vi "Proxy_Build VI Package_vipm_api.vi"(8 "error in (no error)":errorcluster, 10 "Path to VIPB File":path) -> (0 "error out":errorcluster, 2 "Build Output":path)   [LabVIEW 2017, in "CL_G3_VIPMUtilities.lvlib"]
doc: "This VI dynamically invokes the VIPM API with a timeout. VPIM will randomly hang for reasons we don't understand. This vi detects if there is a hang, force closes VIPM and then restarts it."
uses:
  CL_G3_VIPMUtilities.lvlib
  Proxy States.ctl
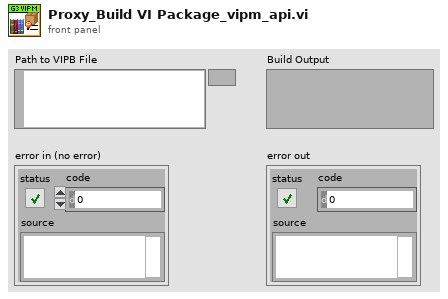
[diagram p1: front panel]
types:
  T1 = typedef "CL_G3_VIPMUtilities.lvlib/Proxy States.ctl" = enum16{"Initialize", "Start Proxy", "Wait on Proxy", "Force Quit VIPM", "Close Proxy"}
  T2 = cluster{"Proxy Path":path, "error out":errorcluster, "Proxy VI Ref":refnum<vi>, "Restart Count":i32, "Maximum restart tries":i32, "Path to VIPB File":path, "Build Output":path}
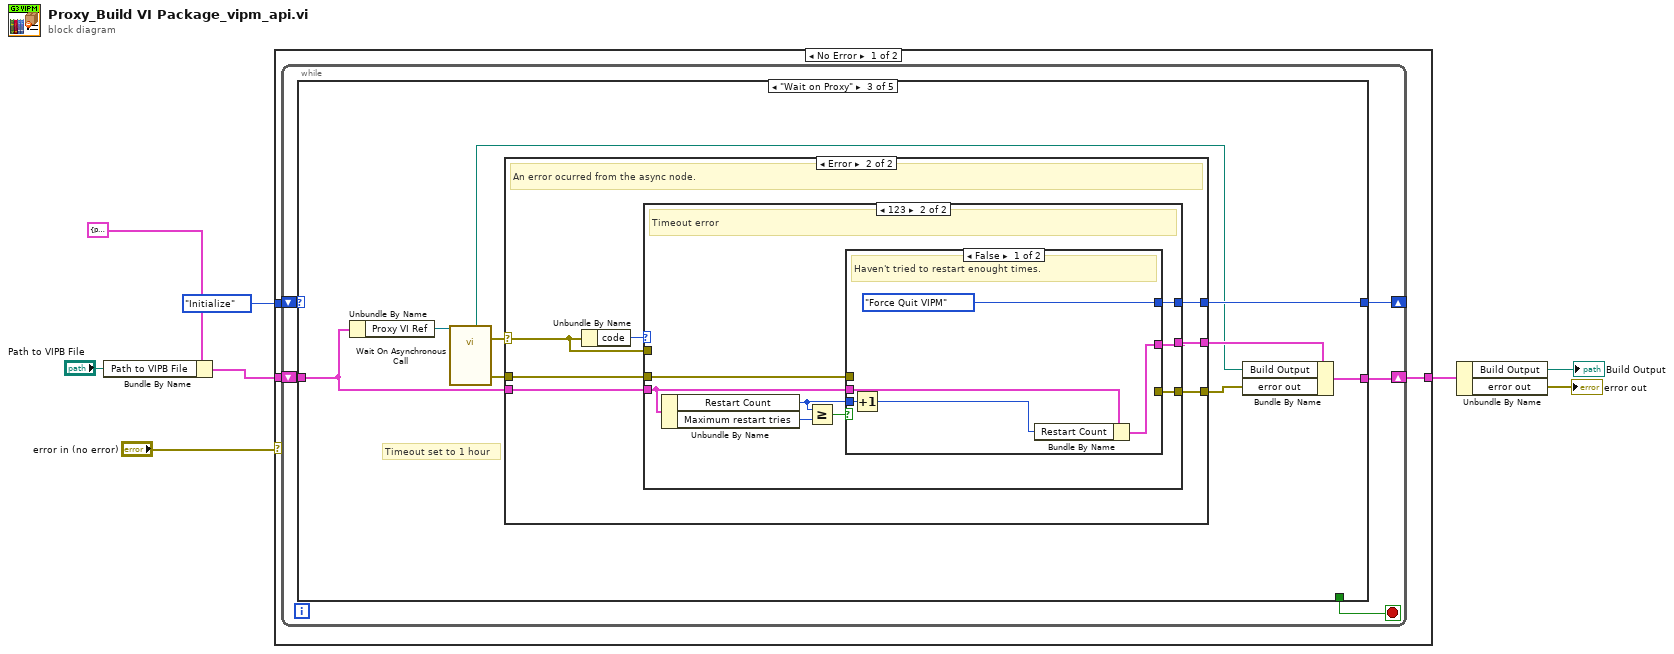
[diagram p0: block diagram]
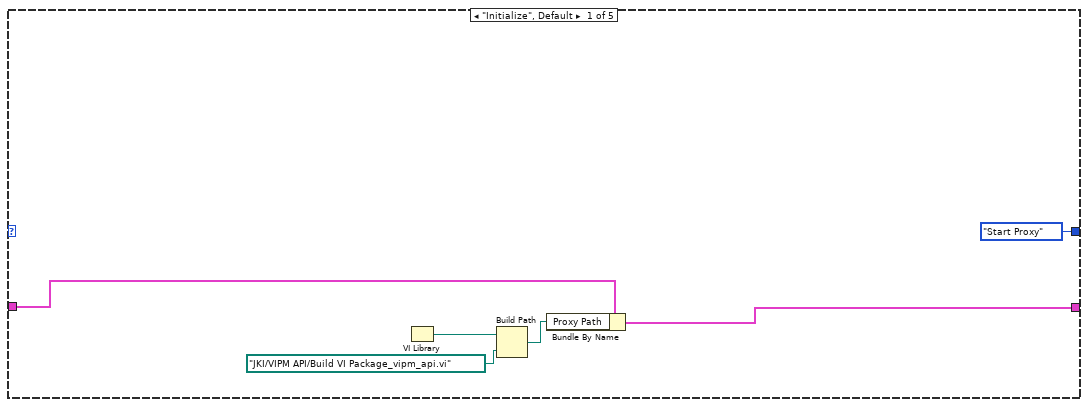
[diagram p2: hidden frame]
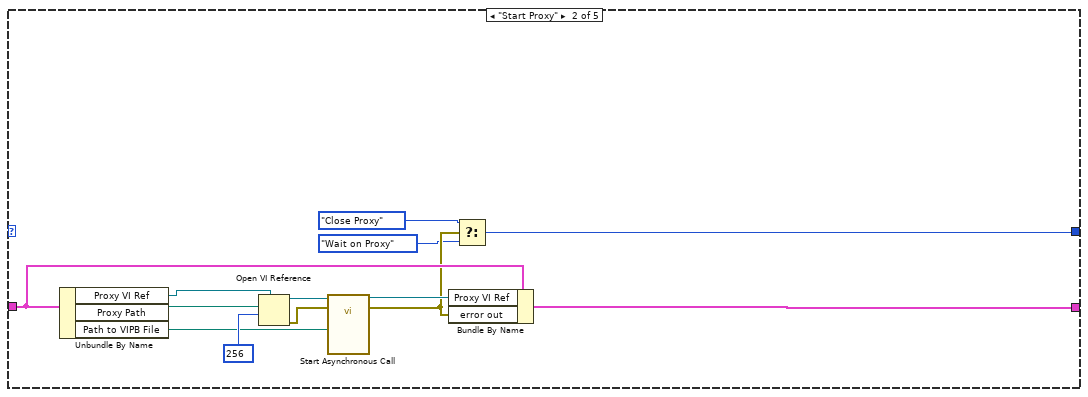
[diagram p3: hidden frame]
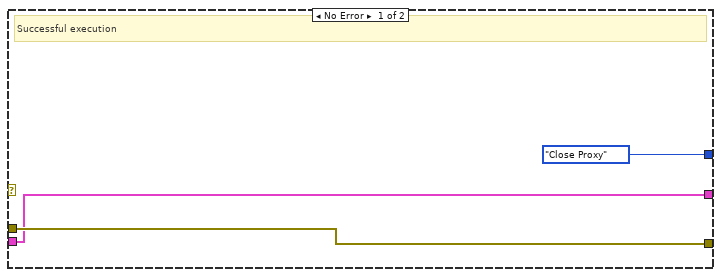
[diagram p4: hidden frame]
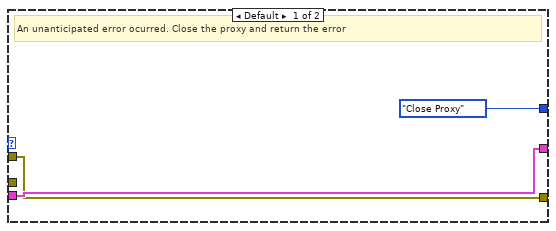
[diagram p5: hidden frame]
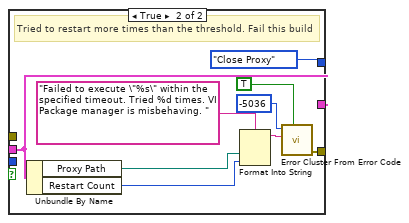
[diagram p6: hidden frame]
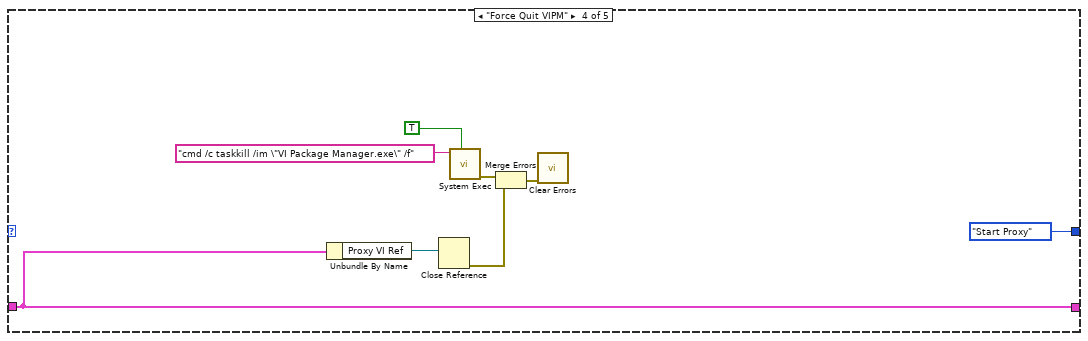
[diagram p7: hidden frame]
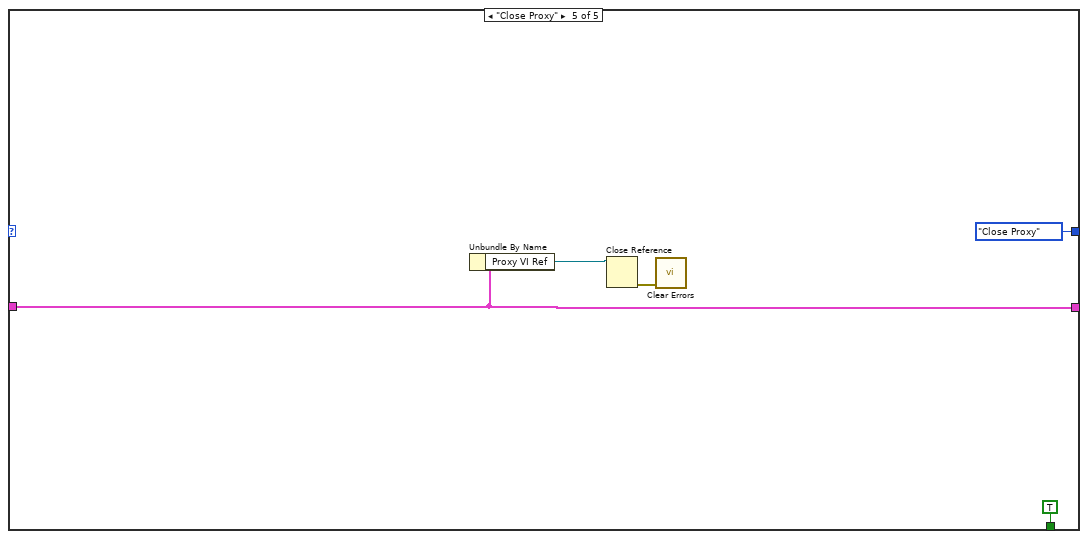
[diagram p8: hidden frame]
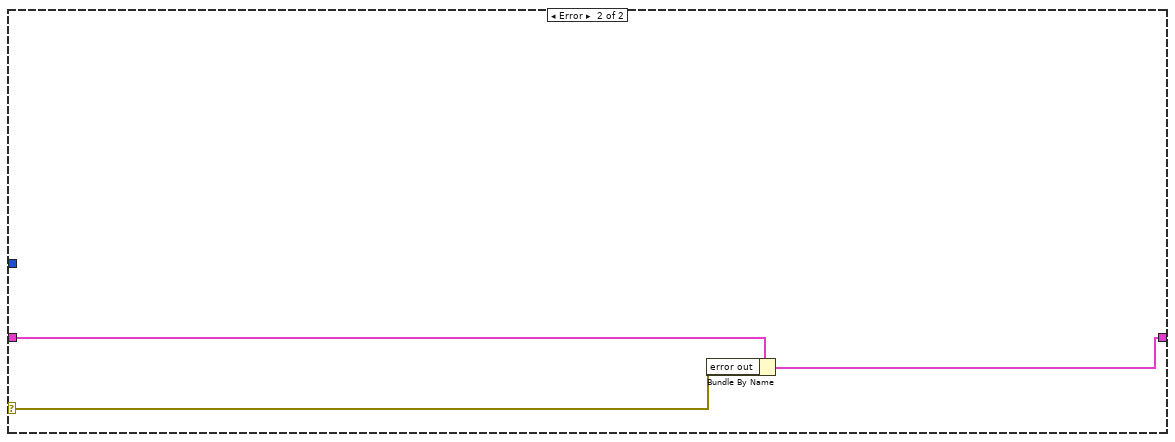
[diagram p9: hidden frame]
diagram:
  n1 = Bundle By Name(cluster=T2 {"Proxy Path"=path "", "error out"={"status"=FALSE, "code"=0, "source"=""}, "Proxy VI Ref"=refnum, "Restart Count"=0, "Maximum restart tries"=5, "Path to VIPB File"=path "", "Build Output"=path ""}, "Path to VIPB File"="Path to VIPB File") -> (w7:T2)
  n2 = case shown="No Error" "error in (no error)" {
    selector: "error in (no error)" -> [_ w94]
    tunnel: w7 -> [w11 w95]
    tunnel: Proxy_States."Initialize" -> [w10 _]
    tunnel: [w9 w93] -> w4
    frame No Error {
      n3 = while {
        shift-right: [w14] -> _
        shift-left: w10 -> [w16]
        shift-right: [w13] -> w9
        shift-left: w11 -> [w15]
        stop <- w12 stop-if-true
        n4 = case shown="\"Wait on Proxy\"" w16 {
          tunnel: [w21 w31 w44 w83 w90] -> w13
          tunnel: w15 -> [w22 w35 w40 w83 w90]
          tunnel: [Proxy_States."Start Proxy" w26 w38 Proxy_States."Start Proxy" Proxy_States."Close Proxy"] -> w14
          tunnel: [_ _ _ _ TRUE] -> w12
          frame "Initialize", Default {
            n5 = VI Library() -> (path=w19:path)
            n6 = Build Path(base path=w19, name or relative path=path "JKI/VIPM API/Build VI Package_vipm_api.vi" ("Proxy Path")) -> (appended path=w17:path)
            n7 = Bundle By Name(cluster=w22, "Proxy Path"=w17) -> (w21:T2)
          }
          frame "Start Proxy" {
            n8 = Unbundle By Name(w35) -> ("Proxy VI Ref"=w25:refnum<vi>, "Proxy Path"=w34:path, "Path to VIPB File"=w23:path)
            n9 = Open VI Reference(type specifier VI Refnum (for type only)=w25, vi path=w34, options=256) -> (vi reference=w33:refnum<vi>, error out=w32:errorcluster)  [unwired: 3 in]
            n10 = call-by-ref "Start Asynchronous Call"(reference=w33, error in=w32, "Path to VIPB File"=w23) -> (reference out=w30:refnum<vi>, error out=w29:errorcluster)  [unwired: 9 in, 2 out]
            n11 = Bundle By Name(cluster=w35, "Proxy VI Ref"=w30, "error out"=w29) -> (w31:T2)
            n12 = Select(t=Proxy_States."Close Proxy", s=w29, f=Proxy_States."Wait on Proxy") -> (s? t:f=w26:T1)
          }
          frame "Wait on Proxy" {
            # "Timeout set to 1 hour"
            n13 = Unbundle By Name(w40) -> ("Proxy VI Ref"=w36:refnum<vi>)
            n14 = call-by-ref "Wait On Asynchronous Call"(reference=w36) -> (error out=w41:errorcluster, 0:"error out"=w42:errorcluster, "Build Output"=w37:path)  [unwired: 11 in, 1 out]
            n15 = case shown="Error" w41 {
              selector: w41 -> [_ w48]
              tunnel: [w47 w51] -> w43
              tunnel: w42 -> [w47 w50]
              tunnel: w40 -> [w45 w53]
              tunnel: [w45 w52] -> w39
              tunnel: [Proxy_States."Close Proxy" w49] -> w38
              frame No Error {
                # "Successful execution"
              }
              frame Error {
                # "An error ocurred from the async node."
                n16 = Unbundle By Name(w48) -> ("code"=w54:i32)
                n17 = case shown="123" w54 {
                  tunnel: w53 -> [w57 w65]
                  tunnel: [w57 w64] -> w52
                  tunnel: [w55 w60] -> w51
                  tunnel: w50 -> [_ w59]
                  tunnel: [Proxy_States."Close Proxy" w61] -> w49
                  tunnel: w48 -> [w55 _]
                  frame Default {
                    # "An unanticipated error ocurred. Close the proxy and return the error"
                  }
                  frame 123 {
                    # "Timeout error"
                    n18 = Unbundle By Name(w65) -> ("Restart Count"=w63:i32, "Maximum restart tries"=w58:i32)
                    n19 = Greater Or Equal?(x=w63, y=w58) -> (x >= y?=w62:bool)
                    n20 = case shown="False" w62 {
                      tunnel: w65 -> [w70 w73]
                      tunnel: [w69 w73] -> w64
                      tunnel: w63 -> [w66 _]
                      tunnel: [Proxy_States."Force Quit VIPM" Proxy_States."Close Proxy"] -> w61
                      tunnel: [_ w77] -> w60
                      tunnel: w59 -> [_ _]
                      frame False {
                        # "Haven't tried to restart enought times."
                        n21 = Increment(x=w66) -> (x+1=w67:i32)
                        n22 = Bundle By Name(cluster=w70, "Restart Count"=w67) -> (w69:T2)
                      }
                      frame True {
                        # "Tried to restart more times than the threshold. Fail this build"
                        n23 = Unbundle By Name(w73) -> ("Proxy Path"=w72:path, "Restart Count"=w71:i32)
                        n24 = Format Into String(format string="Failed to execute \"%s\" within the specified timeout. Tried %d times. VI Package manager is misbehaving. ", w72, w71) -> (resulting string=w74:string)  [unwired: 2 in, 1 out]
                        n25 = call <vilib>:"Error Cluster From Error Code.vi"("show call chain? (False)"=TRUE, "error message (\"\")"=w74, "error code (0)"=-5036) -> ("error out"=w77:errorcluster)  [unwired: 6 in]
                      }
                    }
                  }
                }
              }
            }
            n26 = Bundle By Name(cluster=w39, "Build Output"=w37, "error out"=w43) -> (w44:T2)
          }
          frame "Force Quit VIPM" {
            n27 = Unbundle By Name(w83) -> ("Proxy VI Ref"=w82:refnum<vi>)
            n28 = Close Reference(reference=w82) -> (error out=w80:errorcluster)  [unwired: 1 in]
            n29 = call <vilib>:"System Exec.vi"("run minimized? (F)"=TRUE, "command line"="cmd /c taskkill /im \"VI Package Manager.exe\" /f") -> ("error out"=w85:errorcluster)  [unwired: 6 in, 3 out]
            n30 = Merge Errors(w85, w80) -> (w81:errorcluster)
            n31 = call <vilib>:"Clear Errors.vi"("error in (no error)"=w81) -> ()  [unwired: 5 in, 2 out]
          }
          frame "Close Proxy" {
            n32 = Unbundle By Name(w90) -> ("Proxy VI Ref"=w89:refnum<vi>)
            n33 = Close Reference(reference=w89) -> (error out=w88:errorcluster)  [unwired: 1 in]
            n34 = call <vilib>:"Clear Errors.vi"("error in (no error)"=w88) -> ()  [unwired: 5 in, 2 out]
          }
        }
      }
    }
    frame Error {
      n35 = Bundle By Name(cluster=w95, "error out"=w94) -> (w93:T2)
    }
  }
  n36 = Unbundle By Name(w4) -> ("Build Output"=→"Build Output":path, "error out"=→"error out":errorcluster)
